vi "QMH Create Queue.vi"(7 "Initial Messages":string[](array[string]), 8 "error in (no error)":errorcluster, 11 "Message queue name (unnamed)":string) -> (0 "error out":errorcluster, 3 "queue out":refnum<queue>)   [LabVIEW 2013, in "QHM.lvlib"]
doc: "Create a new event queue or produce a reference to an existing one. Add a list of initial events to the queue."
uses:
  <userlib>/QMH/QMH Add Message to Queue (Array).vi
  QHM.lvlib
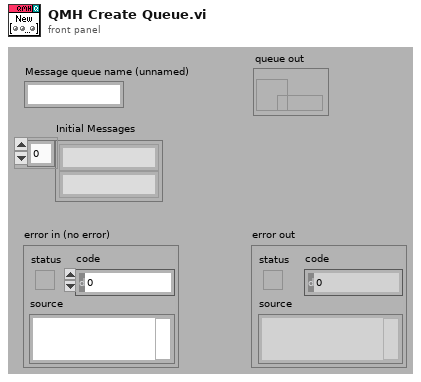
[diagram p1: front panel]
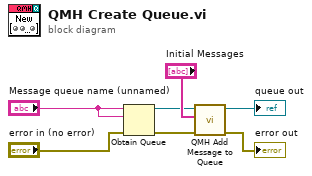
[diagram p0: block diagram]
diagram:
  n1 = Obtain Queue(name (unnamed)="Message queue name (unnamed)", element data type="Message queue name (unnamed)", error in (no error)="error in (no error)") -> (queue out=w1:refnum<queue>, error out=w3:errorcluster)  [unwired: 2 in, 1 out]
  n2 = call-poly <userlib>:"QMH Add Message to Queue.vi"("error in (no error)"=w3, "Messages"="Initial Messages", "queue in"=w1) -> ("error out"=→"error out":errorcluster, "queue out"=→"queue out":refnum<queue>)  [unwired: 7 in]
